vi "RoutedFilterMatch.vi"(8 "error in (no error)":errorcluster, 10 "Filter":T1={"mode"=enum."Mirror", "levelMin"=enum."INFO", "levelMax"=enum."INFO", "tagPrefix"=""}, 11 "Statement":T4={"timestamp"=timestamp(0 s since 1904-01-01), "level"=enum."INFO", "sourceTag"="", "originVI"="", "message"=""}) -> (0 "error out":errorcluster, 3 "Accepted":bool)   [LabVIEW 2026, in "Lumberjack.lvlib"]
doc: "Pure predicate for the routed filter test, evaluating only the Filter control (level band and tag prefix) and assuming the statement has already cleared the appender threshold. accepted is TRUE iff the statement's level is within the inclusive rank band [levelMin, levelMax] AND the sourceTag matches tagPrefix: an empty prefix matches any; a non-empty prefix matches on a dot-hierarchy boundary (app.db matches app.db and app.db.query, not app.database). Does not test the threshold and does not fault. Community."
uses:
  Lumberjack.lvlib
  TypeDefs/Statement.ctl
  TypeDefs/Severity.ctl
  TypeDefs/Filter.ctl
  TypeDefs/FilterMode.ctl
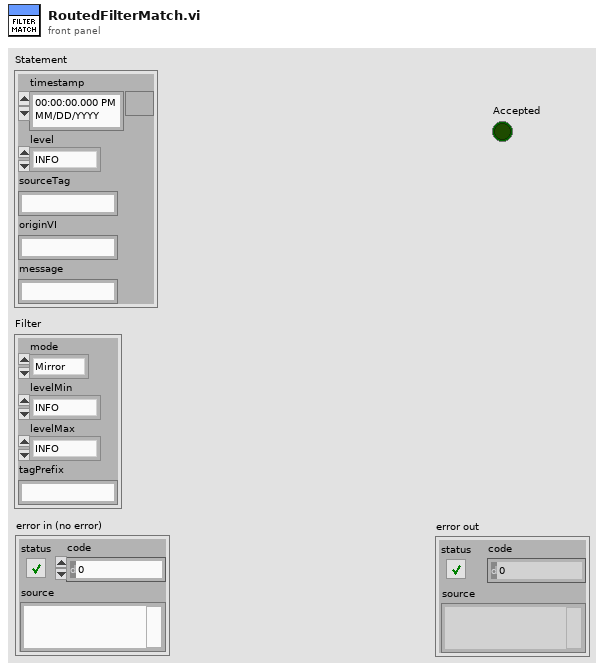
[diagram p1: front panel]
types:
  T1 = typedef "Lumberjack.lvlib/Filter.ctl" = cluster{"mode":T2, "levelMin":T3, "levelMax":T3, "tagPrefix":string}
  T2 = typedef "Lumberjack.lvlib/FilterMode.ctl" = enum16{"Mirror", "Routed"}
  T3 = typedef "Lumberjack.lvlib/Severity.ctl" = enum16{"OFF", "FATAL", "ERROR", "WARN", "INFO", "DEBUG", "TRACE", "ALL"}
  T4 = typedef "Lumberjack.lvlib/Statement.ctl" = cluster{"timestamp":timestamp, "level":T3, "sourceTag":string, "originVI":string, "message":string}
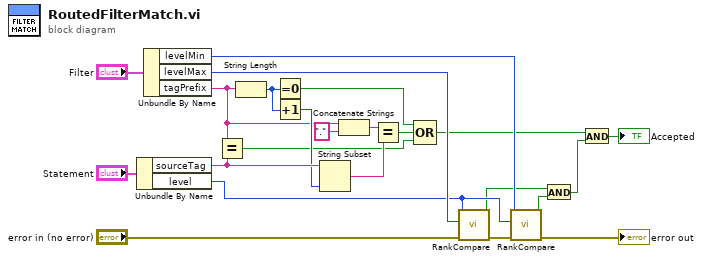
[diagram p0: block diagram]
diagram:
  n1 = Unbundle By Name("Statement") -> ("sourceTag"=w14:string, "level"=w17:T3)
  n2 = Unbundle By Name("Filter") -> ("levelMin"=w18:T3, "levelMax"=w19:T3, "tagPrefix"=w3:string)
  n3 = Equal?(x=w3, y=w14) -> (x = y?=w8:bool)
  n4 = String Length(string=w3) -> (length=w13:i32)
  n5 = Equal To 0?(x=w13) -> (x = 0?=w10:bool)
  n6 = Increment(x=w13) -> (x+1=w12:i32)
  n7 = String Subset(string=w14, length (rest)=w12) -> (substring=w11:string)  [unwired: 1 in]
  n8 = Concatenate Strings(w3, "." ("string")) -> (w1:string)
  n9 = Equal?(x=w1, y=w11) -> (x = y?=w9:bool)
  n10 = Compound Arithmetic op=OR(w10, w9, w8) -> (w6:bool)
  n11 = call "RankCompare.vi"("error in (no error)"="error in (no error)", "Threshold"=w19, "Level"=w17) -> ("error out"=w22:errorcluster, "Passes"=w15:bool)  [unwired: 7 in]
  n12 = call "RankCompare.vi"("error in (no error)"=w22, "Threshold"=w17, "Level"=w18) -> ("error out"=→"error out":errorcluster, "Passes"=w16:bool)  [unwired: 7 in]
  n13 = And(x=w15, y=w16) -> (x .and. y?=w7:bool)
  n14 = And(x=w6, y=w7) -> (x .and. y?=→"Accepted":bool)
